vi "Wait For Device.vi"(6 "Timeout (ms)":i32=20000, 8 "error in":errorcluster) -> (0 "error out":errorcluster, 2 "Success?":bool)   [LabVIEW 2023, in "Application.lvlib"]
uses:
  Application.lvlib
  Resources/GLOBAL/GLOBAL Time-critical.vi
panel:
  out "Waiting time (ms)":i32
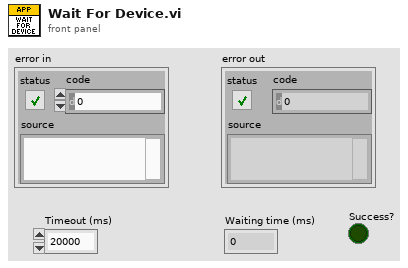
[diagram p1: front panel]
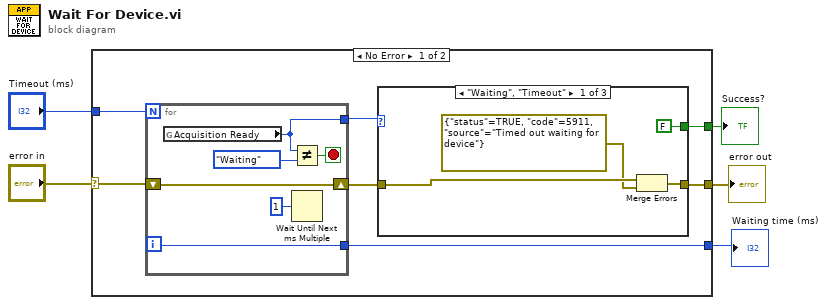
[diagram p0: block diagram]
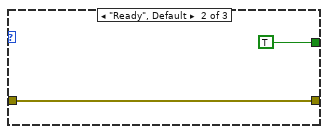
[diagram p2: hidden frame]
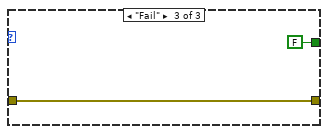
[diagram p3: hidden frame]
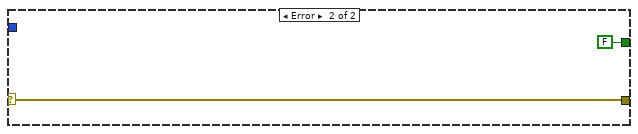
[diagram p4: hidden frame]
diagram:
  n1 = case shown="No Error" "error in" {
    selector: "error in" -> [w11 w28]
    tunnel: "Timeout (ms)" -> [w12 _]
    tunnel: [w10 w28] -> w3
    tunnel: [w8 _] -> w2
    tunnel: [w6 FALSE] -> w1
    frame No Error {
      n2 = for {
        N: w12 -> [_]
        shift-right: [w26] -> w9
        shift-left: w11 -> [w26]
        tunnel: [w22] -> w8
        tunnel: [w21] -> w7
        i -> [w22]
        stop <- w23 stop-if-true
        n3 = global read "GLOBAL Time-critical.vi" "Acquisition Ready"() -> (w21:enum16{"Waiting", "Ready", "Fail", "Timeout"})
        n4 = Not Equal?(x=w21, y=enum16{"Waiting", "Ready", "Fail", "Timeout"}."Waiting") -> (x != y?=w23:bool)
        n5 = Wait Until Next ms Multiple(millisecond multiple=u32 1) -> ()  [unwired: 1 out]
      }
      n6 = case shown="\"Waiting\", \"Timeout\"" w7 {
        tunnel: [w15 w18 w20] -> w10
        tunnel: w9 -> [w14 w18 w20]
        tunnel: [FALSE TRUE FALSE] -> w6
        frame "Waiting", "Timeout" {
          n7 = Merge Errors(w14, errorcluster {"status"=TRUE, "code"=5911, "source"="Timed out waiting for device"} ("error in")) -> (w15:errorcluster)
        }
        frame "Ready", Default {
        }
        frame "Fail" {
        }
      }
    }
    frame Error {
    }
  }
  "error out" <- w3
  "Waiting time (ms)" <- w2
  "Success?" <- w1
